vi "Compare Scalar Clusters.vi"(1 "Target bitfile scalars in":T1[](array[typedef]), 2 "Reference bitfile scalars in":T1[](array[typedef])) -> (0 "Equal ?":bool)   [LabVIEW 2020, in "FPGA Addon Test Class.lvclass"]
uses:
  FPGA Addon Test Class.lvclass
  APIs/Scripting API/TypeDefs/Output Scalar Data.ctl
  Addon/Addon Shared/Types/FPGA Addon Data Type.ctl
  APIs/Scripting API/Scripting API.lvlib
  Addon/Addon Shared/FPGA Addon Shared.lvlib
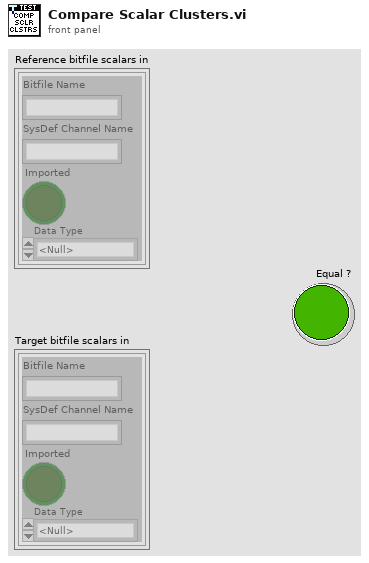
[diagram p1: front panel]
types:
  T1 = typedef "Scripting API.lvlib/Output Scalar Data.ctl" = cluster{"Bitfile Name":string, "SysDef Channel Name":string, "Imported":bool, "Data Type":T2}
  T2 = typedef "FPGA Addon Shared.lvlib/FPGA Addon Data Type.ctl" = enum8{"<Null>", "I8", "I16", "I32", "I64", "U8", "U16", "U32", "U64", "SGL", "Boolean", "Analog PWM In Settings", "Analog PWM In", "Digital PWM In Settings", "Digital PWM In", "Digital PWM Out", "Sine Out", "FXP", "FXP+/-24.5", "FXP+/-16.5", "FXP+/-32.8", "FXP+/-64.32", "FXP+/-16.7", "FXP+/-20.5", "FXP+/-27.5", "FXP+/-32.16", "FXP+16.3", "FXP+18.3", "Digital Static In", "Digital Static Out", "Digital Static In Settings", "Digital WSS Out", "Quad Encoder Settings", "Quad Encoder In", "Group"}
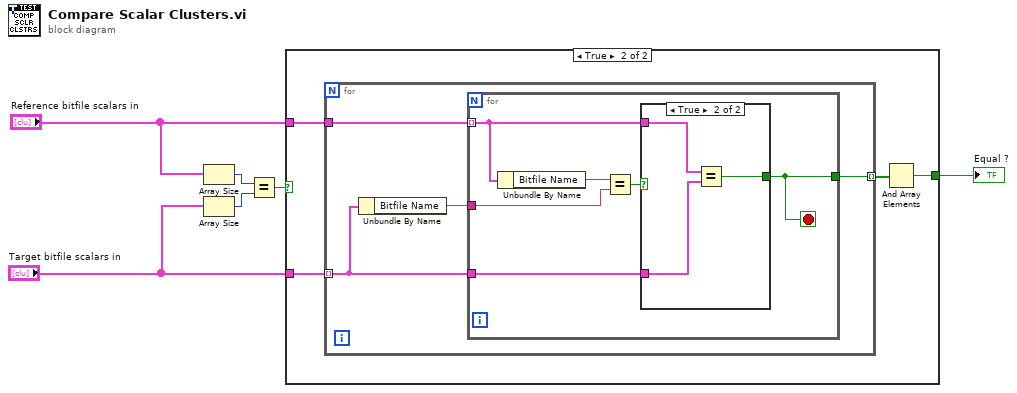
[diagram p0: block diagram]
diagram:
  n1 = Array Size(array="Reference bitfile scalars in") -> (size(s)=w6:i32)
  n2 = Array Size(array="Target bitfile scalars in") -> (size(s)=w5:i32)
  n3 = Equal?(x=w6, y=w5) -> (x = y?=w4:bool)
  n4 = case shown="True" w4 {
    tunnel: "Reference bitfile scalars in" -> [_ w9]
    tunnel: "Target bitfile scalars in" -> [_ w10]
    tunnel: [_ w7] -> w1
    frame False {
    }
    frame True {
      n5 = for {
        tunnel: w10 -> [w12] mode=indexing
        tunnel: w9 -> [w14]
        tunnel: [w11] -> w8 mode=indexing
        n6 = Unbundle By Name(w12) -> ("Bitfile Name"=w13:string)
        n7 = for {
          tunnel: w14 -> [w17] mode=indexing
          tunnel: w13 -> [w19]
          tunnel: w12 -> [w16]
          tunnel: [w15] -> w11
          stop <- w15 stop-if-true
          n8 = Unbundle By Name(w17) -> ("Bitfile Name"=w20:string)
          n9 = Equal?(x=w20, y=w19) -> (x = y?=w18:bool)
          n10 = case shown="True" w18 {
            tunnel: w17 -> [_ w23]
            tunnel: w16 -> [_ w22]
            tunnel: [_ w21] -> w15
            frame False {
            }
            frame True {
              n11 = Equal?(x=w23, y=w22) -> (x = y?=w21:bool)
            }
          }
        }
      }
      n12 = And Array Elements(Boolean array=w8) -> (logical AND=w7:bool)
    }
  }
  "Equal ?" <- w1
